vi "readTableAsString.vi"(8 "error in (no error)":errorcluster, 11 "MS-Excel in":refnum<class "MS-Excel.lvclass">) -> (0 "error out":errorcluster, 2 "Table":string[][](array[string]), 3 "MS-Excel out":refnum<class "MS-Excel.lvclass">)   [LabVIEW 2020, in "LabVIEW NPOI.lvlib" / "MS-Excel.lvclass"]
doc: "Protected dynamic dispatch method to append the wire <b>Table</b> as 2D array of strings to the <b>Document</b> as a table."
uses:
  MS-Excel.lvclass
  D:/Benjamin/Documents/Perso/Code/WC/LabVIEW_NPOI/lib/NPOI 2.1.1/NPOI.dll
  lib/NPOI 2.1.1/NPOI.dll
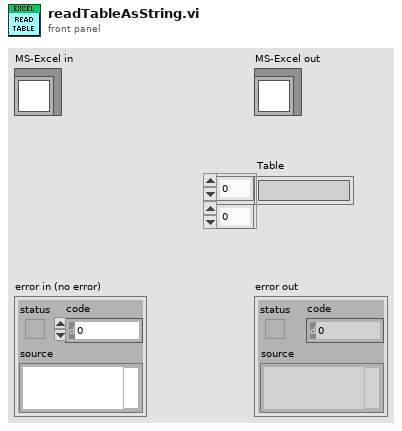
[diagram p1: front panel]
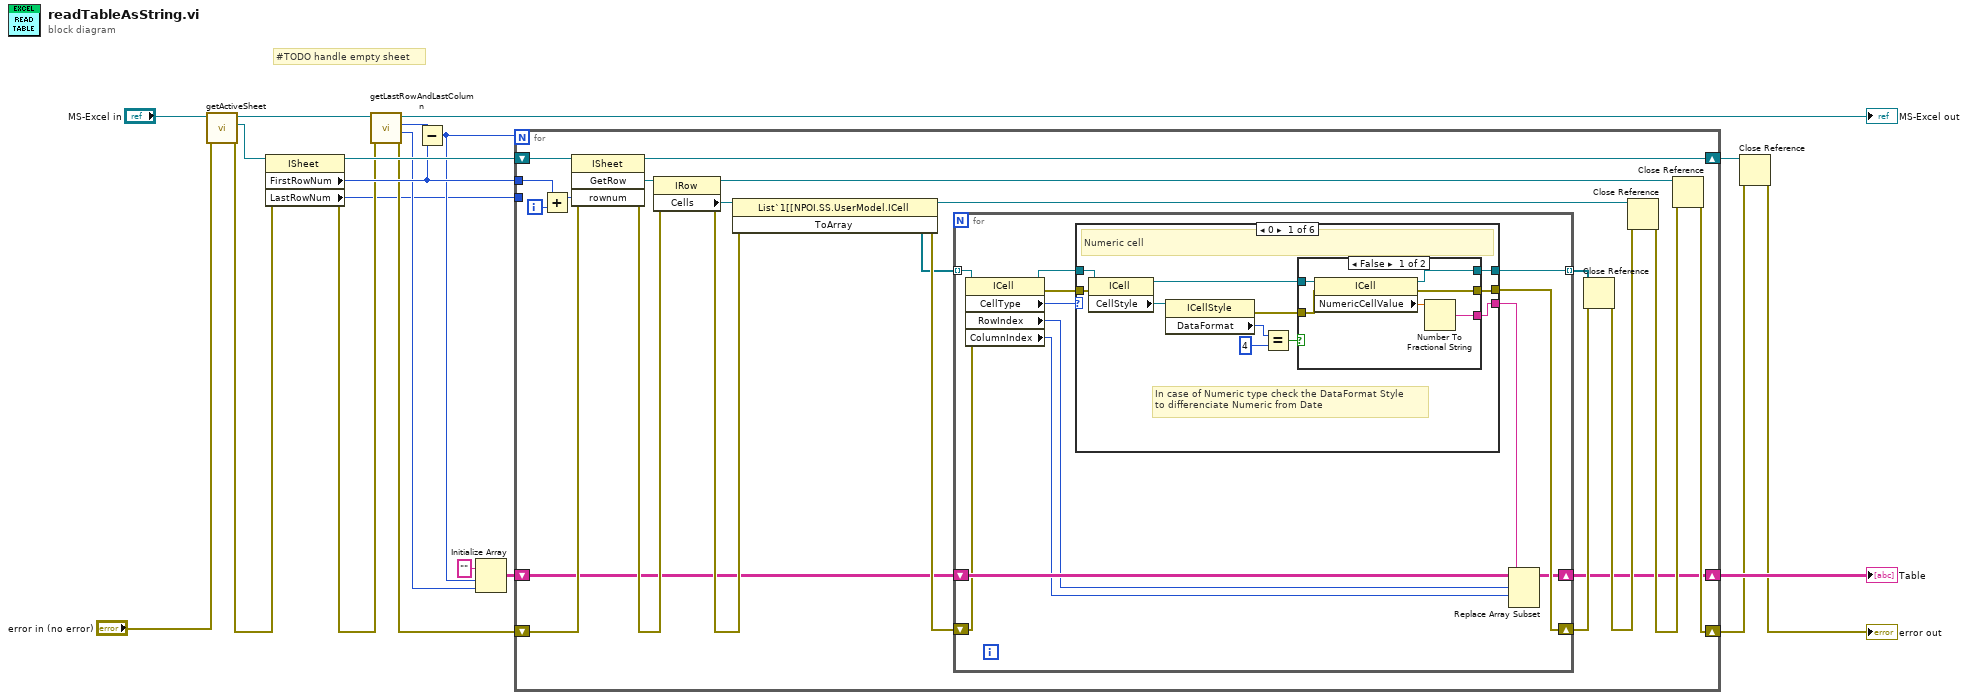
[diagram p0: block diagram]
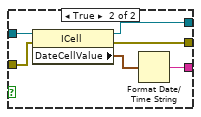
[diagram p2: hidden frame]
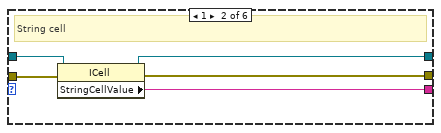
[diagram p3: hidden frame]
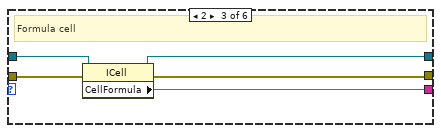
[diagram p4: hidden frame]
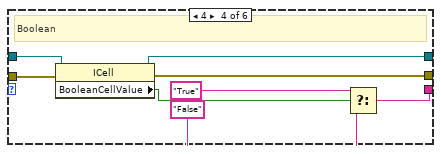
[diagram p5: hidden frame]
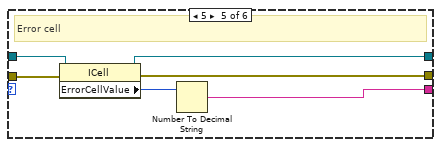
[diagram p6: hidden frame]
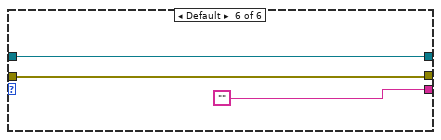
[diagram p7: hidden frame]
diagram:
  # "#TODO handle empty sheet"
  n1 = call-dynamic "getActiveSheet.vi"("error in (no error)"="error in (no error)", "MS-Excel in"="MS-Excel in") -> ("error out"=w17:errorcluster, "Sheet Ref"=w1:refnum<k24>, "MS-Excel out"=w19:refnum<class "MS-Excel.lvclass">)  [unwired: 6 in, 1 out]
  n2 = property class="ISheet"(reference=w1, error in=w17) -> (reference out=w18:refnum<k24>, error out=w7:errorcluster, "FirstRowNum"=w15:i32, "LastRowNum"=w2:i32)
  n3 = call-dynamic "getLastRowAndLastColumn.vi"("error in (no error)"=w7, "MS-Excel in"=w19) -> ("error out"=w6:errorcluster, "Last Column"=w9:i32, "Last Row"=w13:i32, "MS-Excel out"=→"MS-Excel out":refnum<class "MS-Excel.lvclass">)  [unwired: 6 in]
  n4 = Subtract(x=w13, y=w15) -> (x-y=w10:i32)
  n5 = Initialize Array("", w10, w9) -> (w8:string[][])
  n6 = for {
    N: w10 -> [_]
    shift-right: [w31] -> w4
    shift-left: w6 -> [w37]
    tunnel: w15 -> [w34]
    shift-right: [w32] -> w5
    shift-left: w18 -> [w41]
    shift-right: [w24] -> w12
    shift-left: w8 -> [w25]
    tunnel: w2 -> [_]
    i -> [w21]
    n7 = Add(x=w34, y=w21) -> (x+y=w33:i32)
    n8 = invoke class="ISheet" method="GetRow"(reference=w41, error in=w37, "rownum"=w33) -> (reference out=w32:refnum<k24>, error out=w36:errorcluster, "GetRow"=w23:refnum<k24>)  [unwired: 1 in, 1 out]
    n9 = property class="IRow"(reference=w23, error in=w36) -> (reference out=w38:refnum<k24>, error out=w35:errorcluster, "Cells"=w22:refnum<k24>)
    n10 = invoke class="List`1[[NPOI.SS.UserModel.ICell" method="ToArray"(reference=w22, error in=w35) -> (reference out=w40:refnum<k24>, error out=w30:errorcluster, "ToArray"=w29:refnum<k24>[])  [unwired: 1 in]
    n11 = for {
      tunnel: w29 -> [w42] mode=indexing
      shift-right: [w52] -> w27
      shift-left: w30 -> [w45]
      tunnel: [w53] -> w28 mode=indexing
      shift-right: [w48] -> w24
      shift-left: w25 -> [w51]
      n12 = property class="ICell"(reference=w42, error in=w45) -> (reference out=w50:refnum<k24>, error out=w46:errorcluster, "CellType"=w49:i32, "RowIndex"=w44:i32, "ColumnIndex"=w43:i32)
      n13 = case shown="0" w49 {
        tunnel: [w54 w81 w84 w94 w98 w103] -> w53
        tunnel: [w55 w80 w83 w93 w97 w102] -> w52
        tunnel: w50 -> [w61 w79 w86 w92 w100 w103]
        tunnel: [w56 w78 w82 w90 w96 ""] -> w47
        tunnel: w46 -> [w60 w77 w85 w91 w99 w102]
        frame 0 {
          # "In case of Numeric type check the DataFormat Style\nto differenciate Numeric from Date"
          # "Numeric cell"
          n14 = property class="ICell"(reference=w61, error in=w60) -> (reference out=w57:refnum<k24>, "CellStyle"=w64:refnum<k24>)  [unwired: 1 out]
          n15 = property class="ICellStyle"(reference=w64) -> (error out=w58:errorcluster, "DataFormat"=w63:i16)  [unwired: 1 in, 1 out]
          n16 = Equal?(x=w63, y=i16 4) -> (x = y?=w59:bool)
          n17 = case shown="False" w59 {
            tunnel: w58 -> [w69 w75]
            tunnel: w57 -> [w70 w76]
            tunnel: [w67 w73] -> w56
            tunnel: [w65 w72] -> w55
            tunnel: [w66 w71] -> w54
            frame False {
              n18 = property class="ICell"(reference=w70, error in=w69) -> (reference out=w66:refnum<k24>, error out=w65:errorcluster, "NumericCellValue"=w68:dbl)
              n19 = Number To Fractional String(number=w68) -> (F-format string=w67:string)  [unwired: 3 in]
            }
            frame True {
              n20 = property class="ICell"(reference=w76, error in=w75) -> (reference out=w71:refnum<k24>, error out=w72:errorcluster, "DateCellValue"=w74:timestamp)
              n21 = Format Date/Time String(seconds (now)=w74) -> (date/time string=w73:string)  [unwired: 2 in]
            }
          }
        }
        frame 1 {
          # "String cell"
          n22 = property class="ICell"(reference=w79, error in=w77) -> (reference out=w81:refnum<k24>, error out=w80:errorcluster, "StringCellValue"=w78:string)
        }
        frame 2 {
          # "Formula cell"
          n23 = property class="ICell"(reference=w86, error in=w85) -> (reference out=w84:refnum<k24>, error out=w83:errorcluster, "CellFormula"=w82:string)
        }
        frame 4 {
          # "Boolean"
          n24 = property class="ICell"(reference=w92, error in=w91) -> (reference out=w94:refnum<k24>, error out=w93:errorcluster, "BooleanCellValue"=w89:bool)
          n25 = Select(t="True", s=w89, f="False") -> (s? t:f=w90:string)
        }
        frame 5 {
          # "Error cell"
          n26 = property class="ICell"(reference=w100, error in=w99) -> (reference out=w98:refnum<k24>, error out=w97:errorcluster, "ErrorCellValue"=w95:u8)
          n27 = Number To Decimal String(number=w95) -> (decimal integer string=w96:string)  [unwired: 1 in]
        }
        frame Default {
        }
      }
      n28 = Replace Array Subset(array=w51, new element=w47, index (row)=w44, index (col)=w43) -> (w48:string[][])
    }
    n29 = Close Reference(reference=w28, error in (no error)=w27) -> (error out=w26:errorcluster)
    n30 = Close Reference(reference=w40, error in (no error)=w26) -> (error out=w39:errorcluster)
    n31 = Close Reference(reference=w38, error in (no error)=w39) -> (error out=w31:errorcluster)
  }
  "Table" <- w12
  n32 = Close Reference(reference=w5, error in (no error)=w4) -> (error out=→"error out":errorcluster)
